vi "Multiple Straight Line Moves_no_plateau.vi"() -> ()   [LabVIEW 2014]
doc: "This example shows a single axis straight-line move using the NI SoftMotion Line function block.\n\nNote: You must have the LabVIEW NI SoftMotion Module installed to run this example."
uses:
  <vilib>/Motion/Express/_s/nimc.fb.straightLineMove.startStraightLineMove.axis.modeRelative.0.vi
  <vilib>/Motion/Express/_s/nimc.fb.stopMove.stop.axis.modeDecelerate.vi
  <vilib>/Motion/Express/_s/nimc.fb.read.readExecutionData.axis.vi
  <vilib>/Motion/BlockNode/FB.NIMotion.xnode
panel:
  in  "Sync lag":u32=150
  out "Acceleration (decimicrons/s2)":dbl
  out "Velocity (decimicrons/s)":dbl
  out "Position at Peak (decimicrons)":dbl
  in  "Target Peak Displacement (mm)":dbl=2.0
  in  "Target Pulse Duration (ms)":dbl=1000.0
  out "Single Plot (Array of X,Y Pairs)":cluster{u32[], dbl[]}(graph)
  out "Example Done":bool=TRUE
  out "error out":errorcluster={"status"=FALSE, "code"=77003, "source"="Invoke Node in nimc.fb.straightLineMove.startStraightLineMove.axis.modeAbsolute.0.vi:5060005->Multiple Straight Line Moves.vi"}
  in  "Resource":refnum<k21>="Axis 1"
  # "Computed Inputs"
  # "Target Parameters"
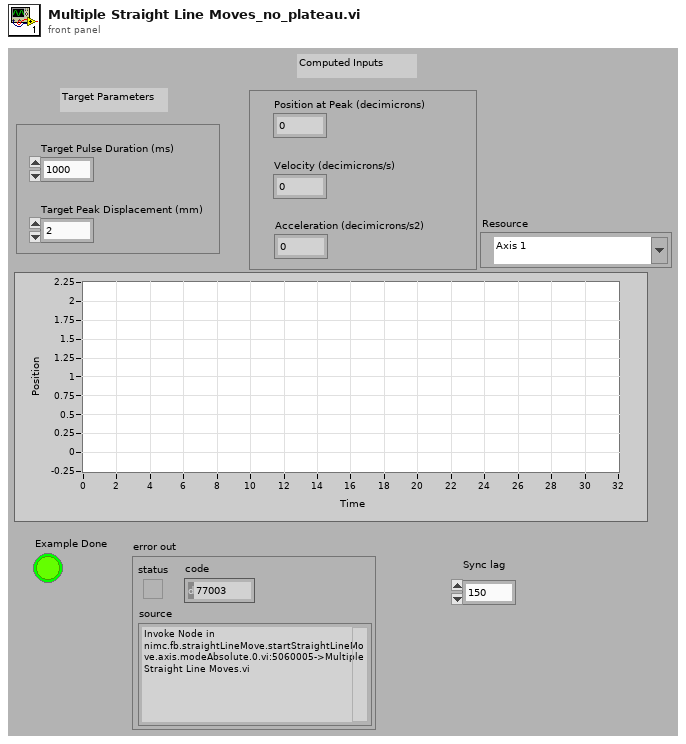
[diagram p1: front panel]
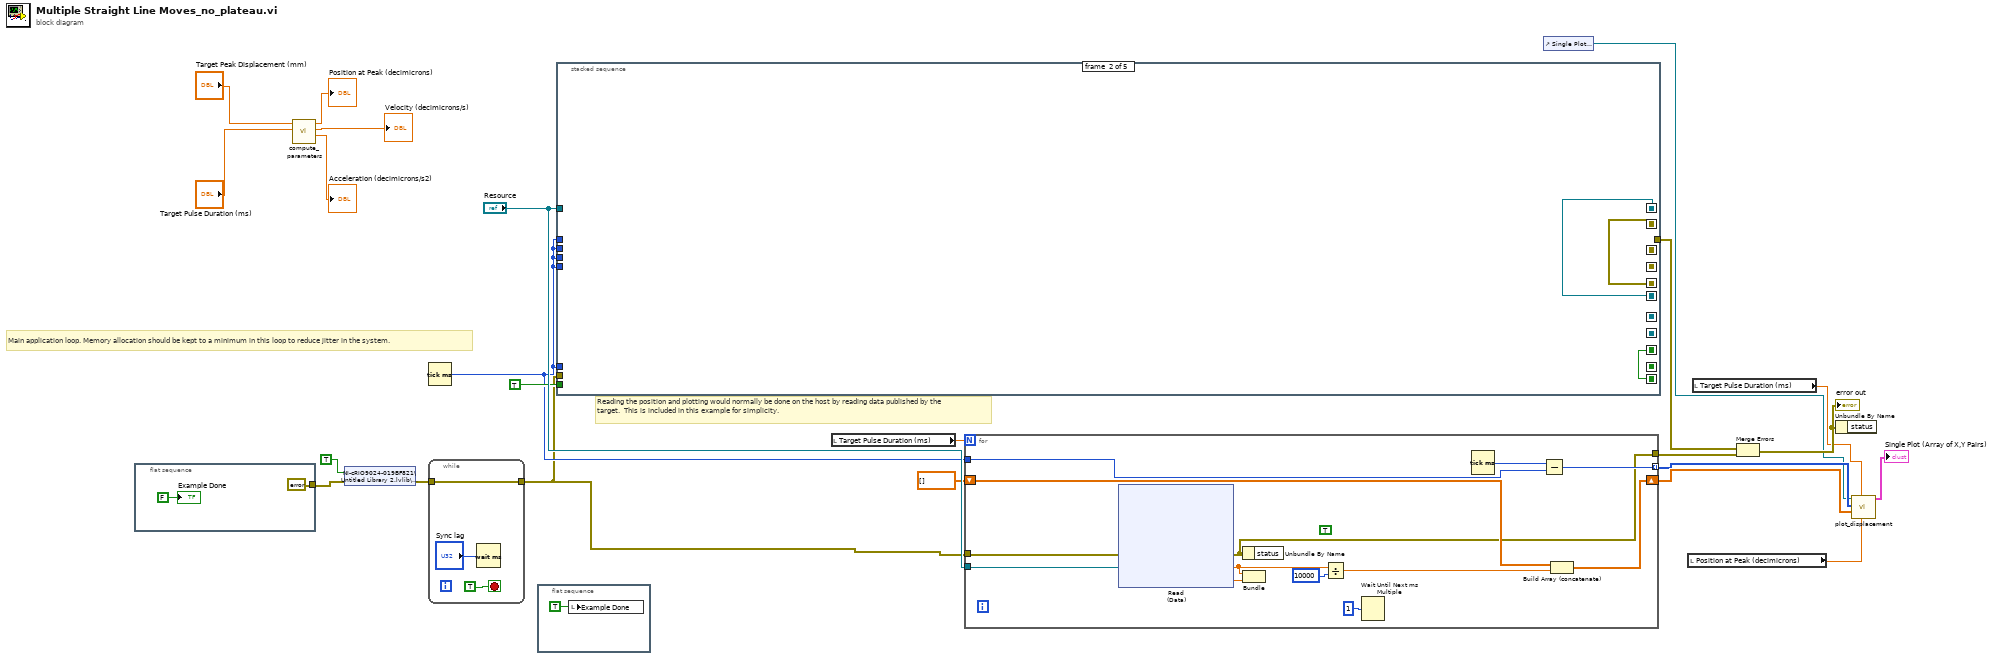
[diagram p0: block diagram]
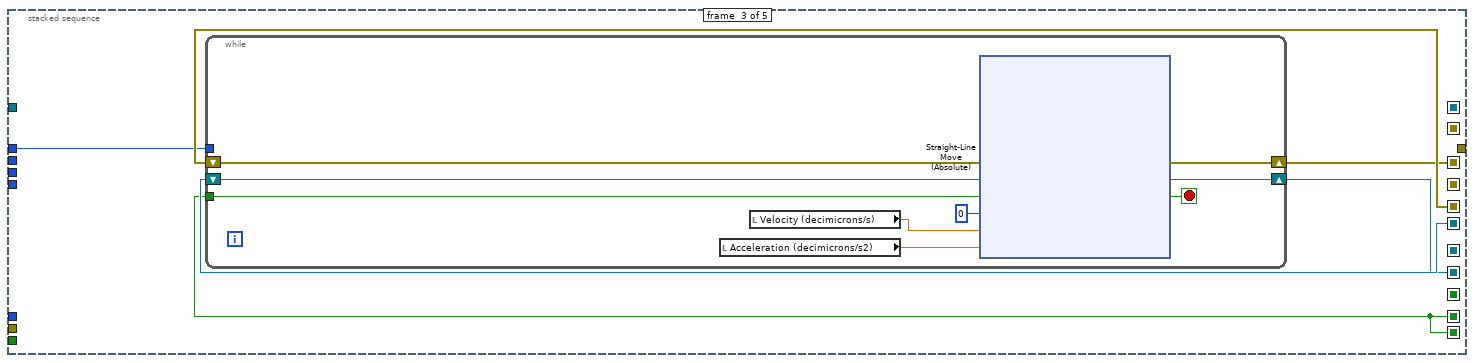
[diagram p3: hidden frame]
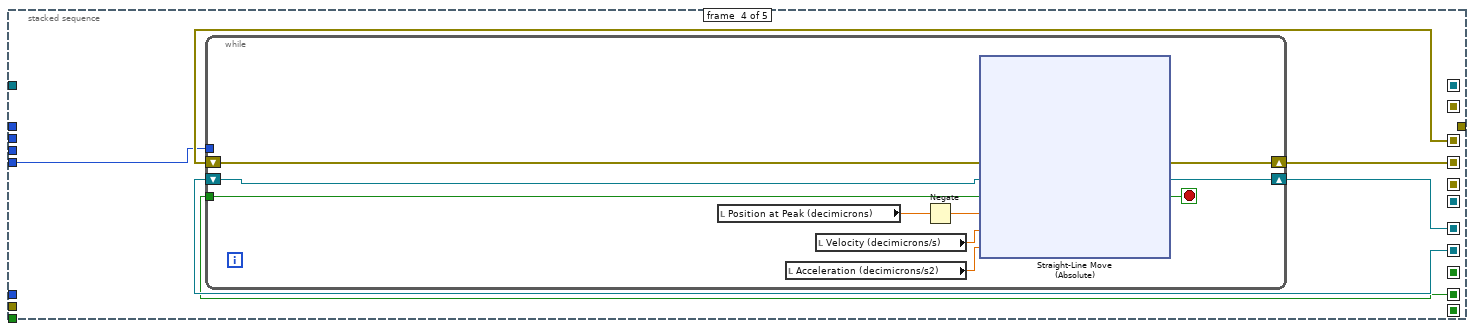
[diagram p4: hidden frame]
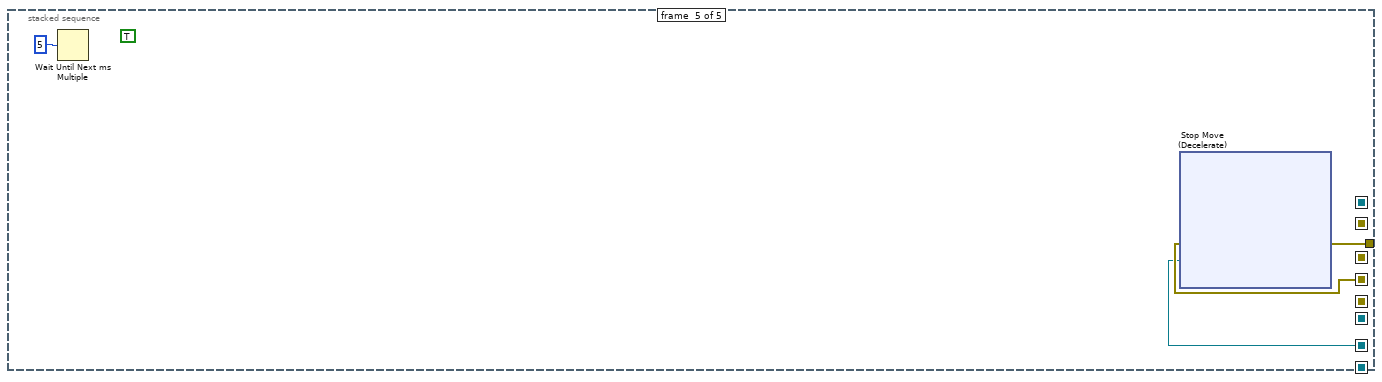
[diagram p5: hidden frame]
diagram:
  # "Reading the position and plotting would normally be done on the host by reading data published by the target.  This is included in this example for simplicity."
  # "Main application loop. Memory allocation should be kept to a minimum in this loop to reduce jitter in the system."
  n1 = flat-sequence {
    tunnel: [errorcluster {"status"=FALSE, "code"=0, "source"=""} ("Error")] -> w3
    frame #0 {
      "Example Done" <- FALSE ("Example Done")
    }
  }
  n2 = call "compute_parameters.vi"("Target Pulse Duration (ms)"="Target Pulse Duration (ms)", "Target Peak Displacement (mm)"="Target Peak Displacement (mm)") -> ("Acceleration (decimicrons/s2)"=→"Acceleration (decimicrons/s2)":dbl, "Velocity (decimicrons/s)"=→"Velocity (decimicrons/s)":dbl, "Position at Peak (decimicrons)"=→"Position at Peak (decimicrons)":dbl)  [unwired: 7 in]
  n3 = shared-variable "NI-cRIO9024-019BF821\\Untitled Library 2.lvlib\\Variable2"(TRUE ("Variable1"), error in=w3) -> (error out=w1:errorcluster)
  n4 = Tick Count (ms)() -> (millisecond timer value=w18:u32)
  n5 = while {
    tunnel: [w26] -> w2
    tunnel: w1 -> [w26]
    stop <- TRUE stop-if-true
    n6 = Wait (ms)(milliseconds to wait="Sync lag") -> ()  [unwired: 1 out]
  }
  n7 = flat-sequence {
    frame #0 {
      n8 = local write "Example Done"(TRUE ("Example Done")) -> ()
    }
  }
  n9 = stacked-sequence {
    seq-local: [w30 _ _ _ _] -> [_ w33 _ _ _]
    seq-local: [w31 _ _ _ _] -> [_ w34 _ _ _]
    seq-local: [w32 _ _ _ _] -> [_ w35 _ _ _]
    seq-local: [_ w33 _ _ _] -> [_ _ w41 _ _]
    seq-local: [_ w34 _ _ _] -> [_ _ w39 _ _]
    seq-local: [_ w35 _ _ _] -> [_ _ w37 _ _]
    seq-local: [_ _ w40 _ _] -> [_ _ _ w73 _]
    seq-local: [_ _ w38 _ _] -> [_ _ _ w71 _]
    seq-local: [_ _ w37 _ _] -> [_ _ _ w69 _]
    seq-local: [_ _ _ w72 _] -> [_ _ _ _ w104]
    seq-local: [_ _ _ w70 _] -> [_ _ _ _ w102]
    tunnel: "Resource" -> [w31 _ _ _ _]
    tunnel: w2 -> [w30 _ _ _ _]
    tunnel: TRUE ("approach forward") -> [w32 _ _ _ _]
    tunnel: w18 -> [_ _ _ _ _]
    tunnel: w18 -> [_ _ _ _ _]
    tunnel: w18 -> [_ _ w36 _ _]
    tunnel: w18 -> [_ _ _ w68 _]
    tunnel: [_ _ _ _ w103] -> w20
    tunnel: w18 -> [_ _ _ _ _]
    frame #0 {
    }
    frame #1 {
    }
    frame #2 {
      n10 = while {
        tunnel: w37 -> [w46]
        tunnel: w36 -> [_]
        shift-right: [w49] -> w40
        shift-left: w41 -> [w50]
        shift-right: [w47] -> w38
        shift-left: w39 -> [w48]
        stop <- w42 stop-if-true
        n11 = local read "Acceleration (decimicrons/s2)"() -> (w44:dbl)
        n12 = local read "Velocity (decimicrons/s)"() -> (w45:dbl)
        n13 = xnode "Straight-Line Move\n(Absolute)"("error in"=w50, "resource"=w48, "execute"=w46, "position"=0, "velocity"=w45, "acceleration"=w44) -> ("error out"=w49:errorcluster, "resource out"=w47:refnum<k21>, "done"=w42:bool)
      }
    }
    frame #3 {
      n14 = while {
        tunnel: w69 -> [w79]
        tunnel: w68 -> [_]
        shift-right: [w82] -> w72
        shift-left: w73 -> [w83]
        shift-right: [w80] -> w70
        shift-left: w71 -> [w81]
        stop <- w74 stop-if-true
        n15 = local read "Position at Peak (decimicrons)"() -> (w76:dbl)
        n16 = local read "Acceleration (decimicrons/s2)"() -> (w77:dbl)
        n17 = local read "Velocity (decimicrons/s)"() -> (w78:dbl)
        n18 = Negate(x=w76) -> (-x=w75:dbl)
        n19 = xnode "Straight-Line Move\n(Absolute)"("error in"=w83, "resource"=w81, "execute"=w79, "position"=w75, "velocity"=w78, "acceleration"=w77) -> ("error out"=w82:errorcluster, "resource out"=w80:refnum<k21>, "done"=w74:bool)
      }
    }
    frame #4 {
      (unwired) TRUE
      n20 = Wait Until Next ms Multiple(millisecond multiple=u32 5) -> ()  [unwired: 1 out]
      n21 = xnode "Stop Move\n(Decelerate)"("error in"=w104, "resource"=w102) -> ("error out"=w103:errorcluster)  [unwired: 1 in, 1 out]
    }
  }
  n22 = local read "Target Pulse Duration (ms)"() -> (w16:dbl)
  n23 = for {
    N: w16 -> [_]
    tunnel: "Resource" -> [w123]
    tunnel: w2 -> [w124]
    tunnel: [w112] -> w22
    tunnel: w18 -> [w120]
    shift-right: [w116] -> w8
    shift-left: dbl[] [] -> [w117]
    tunnel: [w113] -> w7 mode=indexing
    (unwired) TRUE ("Variable2")
    n24 = xnode "Read\n(Data)"("error in"=w124, "resource"=w123) -> ("error out"=w112:errorcluster, "position"=w118:dbl, "velocity"=w122:dbl)
    n25 = Unbundle By Name(w112) -> ()  [unwired: 1 out]
    n26 = Bundle("position"=w118, "velocity"=w122) -> ()  [unwired: 2 out]
    n27 = Divide(x=w118, y=10000) -> (x/y=w115:dbl)
    n28 = Wait Until Next ms Multiple(millisecond multiple=u32 1) -> ()  [unwired: 1 out]
    n29 = Tick Count (ms)() -> (millisecond timer value=w121:u32)
    n30 = Subtract(x=w121, y=w120) -> (x-y=w113:u32)
    n31 = Build Array (concatenate)(w117, w115) -> (w116:dbl[])
  }
  n32 = control-ref of="Single Plot (Array of X,Y Pairs)"() -> (w5:refnum<vi>)
  n33 = local read "Position at Peak (decimicrons)"() -> (w9:dbl)
  n34 = local read "Target Pulse Duration (ms)"() -> (w6:dbl)
  n35 = Merge Errors(w20, w22) -> (w19:errorcluster)
  "error out" <- w19
  n36 = Unbundle By Name(w19) -> ()  [unwired: 1 out]
  n37 = call "plot_displacement.vi"("Position at Peak (decimicrons)"=w9, "Target Pulse Duration (ms)"=w6, "Array"=w8, "Array 2"=w7, "XYGraph in"=w5) -> ("Cluster"=→"Single Plot (Array of X,Y Pairs)":cluster{u32[], dbl[]})  [unwired: 6 in]
